vi "Clean Up Wires on New Objects.vi"(8 "error in (no error)":errorcluster, 11 "New objects created":refnum<vi>[](array[refnum])) -> (0 "error out":errorcluster)   [LabVIEW 2023]
doc: "clean up wires on newly created objects."
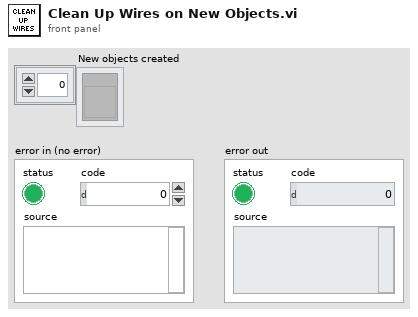
[diagram p1: front panel]
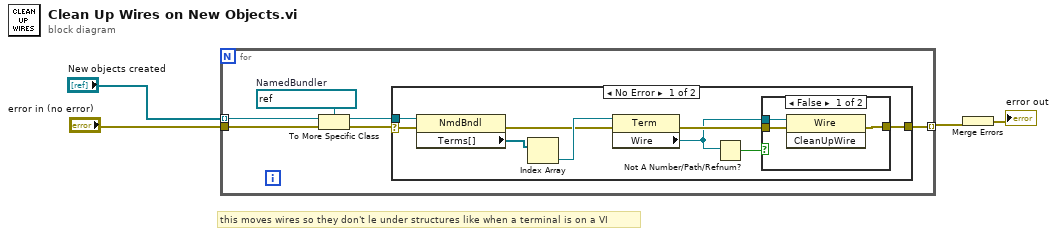
[diagram p0: block diagram]
diagram:
  # "this moves wires so they don't le under structures like when a terminal is on a VI"
  n1 = for {
    tunnel: "New objects created" -> [w7] mode=indexing
    tunnel: [w6] -> w3 mode=indexing
    tunnel: "error in (no error)" -> [w5]
    w9 = refnum<vi> refnum  # NamedBundler
    n2 = To More Specific Class(target class=w9, reference=w7, error in=w5) -> (specific class reference=w10:refnum<vi>, error out=w8:errorcluster)
    n3 = case shown="No Error" w8 {
      selector: w8 -> [w17 _]
      tunnel: w10 -> [w19 _]
      tunnel: [w16 _] -> w6
      frame No Error {
        n4 = property class="NmdBndl"(reference=w19, error in=w17) -> (error out=w14:errorcluster, "Terms[]"=w18:refnum<vi>[])  [unwired: 1 out]
        n5 = Index Array(array=w18) -> (element=w15:refnum<vi>)  [unwired: 1 in]
        n6 = property class="Term"(reference=w15, error in=w14) -> (error out=w13:errorcluster, "Wire"=w12:refnum<vi>)  [unwired: 1 out]
        n7 = Not A Number/Path/Refnum?(number/path/refnum=w12) -> (NaN/Path/Refnum?=w11:bool)
        n8 = case shown="False" w11 {
          tunnel: [w22 w23] -> w16
          tunnel: w12 -> [w21 _]
          tunnel: w13 -> [w20 w23]
          frame False {
            n9 = invoke class="Wire" method="CleanUpWire"(reference=w21, error in=w20) -> (error out=w22:errorcluster)  [unwired: 1 in, 2 out]
          }
          frame True {
          }
        }
      }
      frame Error {
      }
    }
  }
  n10 = Merge Errors(w3) -> (→"error out":errorcluster)
